vi "View DO param.vi"(7 "ActivateDIView":bool, 9 "DO in":T1, 10 "DO_State":T2[](array[typedef]), 11 "DOTable":bool[](array[boolean])) -> (2 "Reread out":bool, 3 "This VI":refnum<vi>)   [LabVIEW 2019, in "Inputs.lvlib"]
uses:
  Inputs.lvlib
  Ctl/Parameter State.ctl
  Ctl/DO.ctl
  Database/Progress.vi
  Database/PostgreSQL.lvlib
  Logik/Logik.lvlib
panel:
  out "DO9":bool
  out "DO8":bool
  out "DO7":bool
  out "DO6":bool
  out "DO5":bool
  out "DO4":bool
  out "DO3":bool
  out "DO2":bool
  out "DO1":bool
  out "DO0":bool
  out "DO progress":i32(slide) scale=0.0..100.0
  in  "Reread":bool
  in  "n_elem":i32(c297)
  out "n param":i32
  out "Names table":string[](array[string])
  out "parameters":string[](array[string])
  out "Parameters table":dbl[][](array[numeric])
  # "control_channel_num"
  # "module_num"
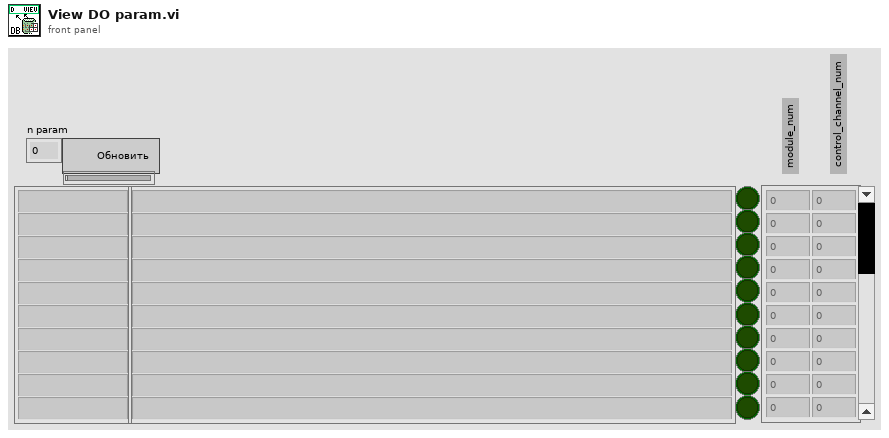
[diagram p1: front panel]
types:
  T1 = typedef "Inputs.lvlib/DO.ctl" = cluster{"DO_defs":cluster{"DO_def":bool[], "DO2D_def":bool[][], "DOState_def":T2[], "DOALRState_def":errorcluster[]}, "modified":refnum<data-value>, "DOP":refnum<data-value>, "DONames":refnum<data-value>}
  T2 = typedef "Inputs.lvlib/Parameter State.ctl" = cluster{"code":i32, "visible":bool, "color":u32, "source":string}
  T3 = enum32{"Invalid", "Standard", "Closed", "Hidden", "Minimized", "Maximized"}
  T4 = enum8{"Enabled", "Disabled", "Disabled and Grayed Out"}
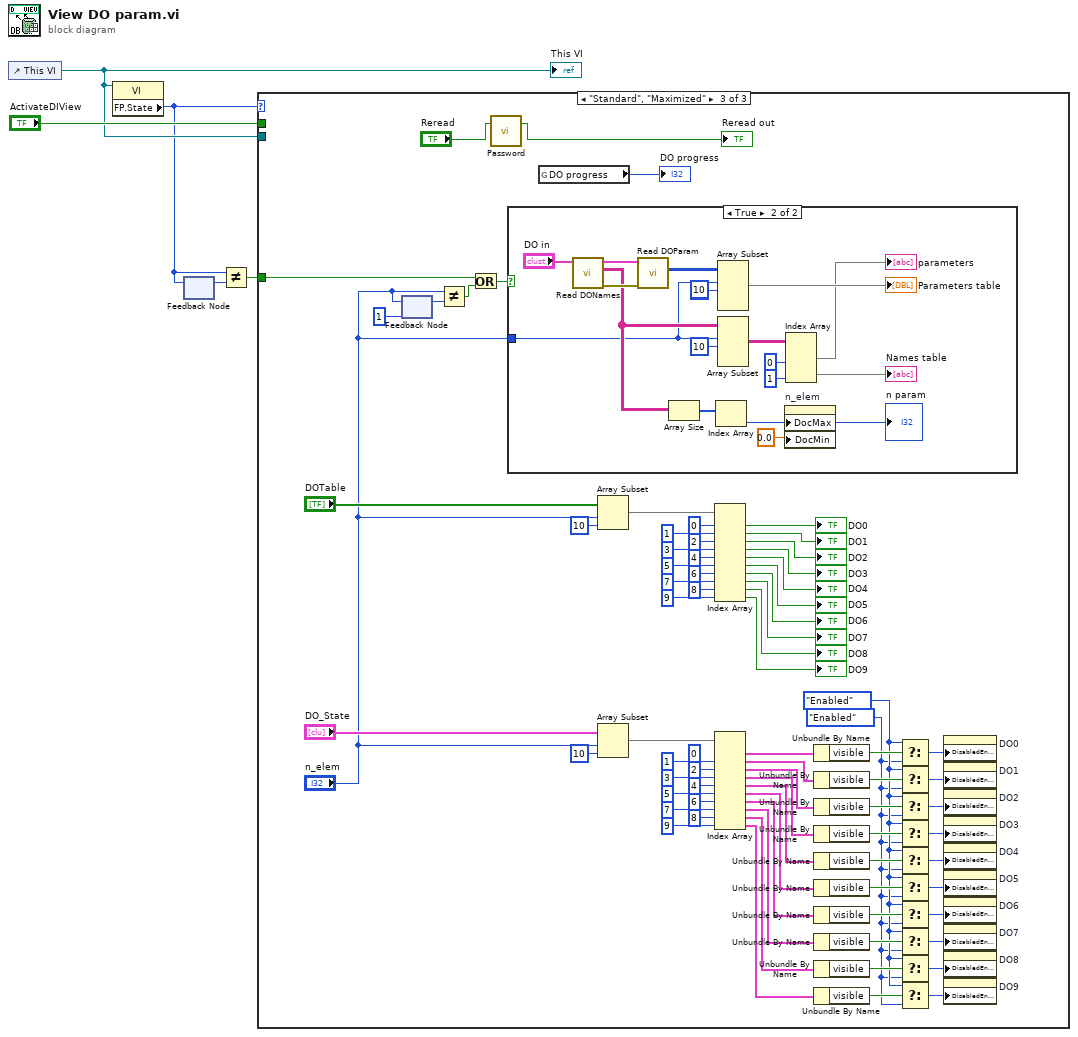
[diagram p0: block diagram]
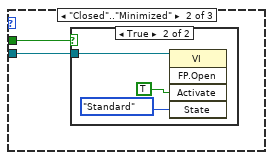
[diagram p3: hidden frame]
diagram:
  n1 = control-ref of="This VI"() -> (w4:refnum<vi>)
  "This VI" <- w4
  n2 = property class="VI"(reference=w4) -> ("FP.State"=w1:T3)  [unwired: 1 in, 2 out]
  n3 = feedback #1() -> (w3:T3)  [unwired: 1 in]
  n4 = feedback-in #1(w1) -> ()
  n5 = Not Equal?(x=w1, y=w3) -> (x != y?=w2:bool)
  n6 = case shown="\"Standard\", \"Maximized\"" w1 {
    tunnel: "ActivateDIView" -> [_ w7 _]
    tunnel: w4 -> [_ w6 _]
    tunnel: w2 -> [_ _ w11]
    frame "Invalid", Default {
    }
    frame "Closed".."Minimized" {
      n7 = case shown="True" w7 {
        tunnel: w6 -> [_ w8]
        frame False {
        }
        frame True {
          n8 = invoke class="VI" method="FP.Open"(reference=w8, "Activate"=TRUE ("Activate?"), "State"=T3."Standard") -> ()  [unwired: 2 in, 5 out]
        }
      }
    }
    frame "Standard", "Maximized" {
      (unwired) 0 ("index")
      w20 = T4."Enabled" ("Disabled")
      w19 = T4."Enabled" ("Disabled")
      n9 = feedback #2(1 ("n_elem")) -> (w16:i32)
      n10 = feedback-in #2("n_elem") -> ()
      n11 = Not Equal?(x="n_elem", y=w16) -> (x != y?=w15:bool)
      n12 = Or(x=w11, y=w15) -> (x .or. y?=w13:bool)
      n13 = call "Password.vi"("ActivatePASSWView"="Reread") -> ("enable"=→"Reread out":bool)  [unwired: 1 in, 1 out]
      n14 = case shown="True" w13 {
        tunnel: "n_elem" -> [_ w87]
        frame False {
        }
        frame True {
          (unwired) 10 ("length")
          n15 = call "Read DONames.vi"("DO in"="DO in") -> ("error out"=w93:errorcluster, "DONames"=w90:string[][], "DO out"=w95:T1)  [unwired: 8 in]
          n16 = call "Read DOParam.vi"("error in (no error)"=w93, "DO in"=w95) -> ("DOParam"=w94:i32[][])  [unwired: 7 in, 2 out]
          n17 = Array Size(array=w90) -> (size(s)=w96:i32[])
          n18 = Index Array(array=w96) -> (element=w89:i32)  [unwired: 1 in]
          "n param" <- w89
          n19 = Array Subset(array=w94, index (row)=w87, length (row)=10 ("length")) -> (→"Parameters table":i32[][])  [unwired: 2 in]
          n20 = Array Subset(array=w90, index (row)=w87, length (row)=10 ("length")) -> (w97:string[][])  [unwired: 2 in]
          n21 = property on="n_elem" class="Scroll (strict)"("DocMax"=w89, "DocMin"=0.0 ("Data Entry Limits:Minimum")) -> ()  [unwired: 2 in, 2 out]
          n22 = Index Array(array=w97, index (col) #1=0 ("disabled index (col)"), index (col) #2=1 ("disabled index (col)")) -> (element #1=→"parameters":string[], element #2=→"Names table":string[])  [unwired: 2 in]
        }
      }
      n23 = global read "Progress.vi" "DO progress"() -> (→"DO progress":i32)
      n24 = Array Subset(array="DOTable", index="n_elem", length=10) -> (w73:bool[])
      n25 = Array Subset(array="DO_State", index="n_elem", length=10) -> (w51:T2[])
      n26 = Index Array(array=w73, index #1=0 ("index"), index #2=1 ("index"), index #3=2 ("index"), index #4=3 ("index"), index #5=4 ("index"), index #6=5 ("index"), index #7=6 ("index"), index #8=7 ("index"), index #9=8 ("index"), index #10=9 ("index")) -> (element #1=→"DO0":bool, element #2=→"DO1":bool, element #3=→"DO2":bool, element #4=→"DO3":bool, element #5=→"DO4":bool, element #6=→"DO5":bool, element #7=→"DO6":bool, element #8=→"DO7":bool, element #9=→"DO8":bool, element #10=→"DO9":bool)
      n27 = Index Array(array=w51, index #2=1 ("index"), index #3=2 ("index"), index #4=3 ("index"), index #5=4 ("index"), index #6=5 ("index"), index #7=6 ("index"), index #8=7 ("index"), index #9=8 ("index"), index #10=9 ("index")) -> (element #1=w50:T2, element #2=w21:T2, element #3=w22:T2, element #4=w23:T2, element #5=w24:T2, element #6=w25:T2, element #7=w26:T2, element #8=w27:T2, element #9=w28:T2, element #10=w29:T2)  [unwired: 1 in]
      n28 = Unbundle By Name(w50) -> ("visible"=w49:bool)
      n29 = Unbundle By Name(w21) -> ("visible"=w46:bool)
      n30 = Unbundle By Name(w22) -> ("visible"=w45:bool)
      n31 = Unbundle By Name(w23) -> ("visible"=w42:bool)
      n32 = Unbundle By Name(w24) -> ("visible"=w41:bool)
      n33 = Unbundle By Name(w25) -> ("visible"=w38:bool)
      n34 = Unbundle By Name(w26) -> ("visible"=w37:bool)
      n35 = Unbundle By Name(w27) -> ("visible"=w35:bool)
      n36 = Unbundle By Name(w28) -> ("visible"=w33:bool)
      n37 = Unbundle By Name(w29) -> ("visible"=w32:bool)
      n38 = Select(t=w20, s=w49, f=w19) -> (s? t:f=w48:T4)
      n39 = Select(t=w20, s=w46, f=w19) -> (s? t:f=w47:T4)
      n40 = Select(t=w20, s=w45, f=w19) -> (s? t:f=w44:T4)
      n41 = Select(t=w20, s=w42, f=w19) -> (s? t:f=w43:T4)
      n42 = Select(t=w20, s=w41, f=w19) -> (s? t:f=w40:T4)
      n43 = Select(t=w20, s=w38, f=w19) -> (s? t:f=w39:T4)
      n44 = Select(t=w20, s=w37, f=w19) -> (s? t:f=w36:T4)
      n45 = Select(t=w20, s=w35, f=w19) -> (s? t:f=w34:T4)
      n46 = Select(t=w20, s=w33, f=w19) -> (s? t:f=w31:T4)
      n47 = Select(t=w20, s=w32, f=w19) -> (s? t:f=w30:T4)
      n48 = property on="DO0" class="Bool (strict)"("DisabledEnum"=w48) -> ()  [unwired: 2 in, 2 out]
      n49 = property on="DO1" class="Bool (strict)"("DisabledEnum"=w47) -> ()  [unwired: 2 in, 2 out]
      n50 = property on="DO2" class="Bool (strict)"("DisabledEnum"=w44) -> ()  [unwired: 2 in, 2 out]
      n51 = property on="DO3" class="Bool (strict)"("DisabledEnum"=w43) -> ()  [unwired: 2 in, 2 out]
      n52 = property on="DO4" class="Bool (strict)"("DisabledEnum"=w40) -> ()  [unwired: 2 in, 2 out]
      n53 = property on="DO5" class="Bool (strict)"("DisabledEnum"=w39) -> ()  [unwired: 2 in, 2 out]
      n54 = property on="DO6" class="Bool (strict)"("DisabledEnum"=w36) -> ()  [unwired: 2 in, 2 out]
      n55 = property on="DO7" class="Bool (strict)"("DisabledEnum"=w34) -> ()  [unwired: 2 in, 2 out]
      n56 = property on="DO8" class="Bool (strict)"("DisabledEnum"=w31) -> ()  [unwired: 2 in, 2 out]
      n57 = property on="DO9" class="Bool (strict)"("DisabledEnum"=w30) -> ()  [unwired: 2 in, 2 out]
    }
  }
